vi "GetLIDARObstacles.vi"(11 "LIDAR data":cluster{"Magnitude":dbl[], "Direction":dbl[]}) -> (3 "LIDAR obstacles":cluster{dbl[], dbl[], i32})   [LabVIEW 2011]
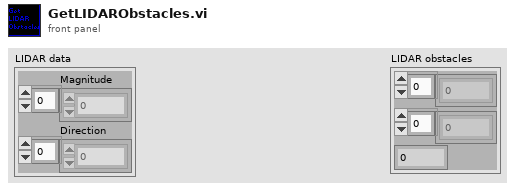
[diagram p1: front panel]
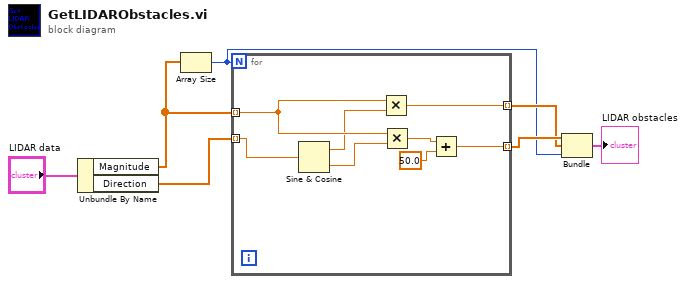
[diagram p0: block diagram]
diagram:
  n1 = Unbundle By Name("LIDAR data") -> ("Magnitude"=w7:dbl[], "Direction"=w6:dbl[])
  n2 = Array Size(array=w7) -> (size(s)=w3:i32)
  n3 = for {
    N: w3 -> [_]
    tunnel: w7 -> [w14] mode=indexing
    tunnel: w6 -> [w15] mode=indexing
    tunnel: [w11] -> w4 mode=indexing
    tunnel: [w8] -> w5 mode=indexing
    n4 = Sine & Cosine(0:w15) -> (1:w13:dbl, 2:w12:dbl)
    n5 = Multiply(x=w14, y=w13) -> (x*y=w11:dbl)
    n6 = Multiply(x=w14, y=w12) -> (x*y=w10:dbl)
    n7 = Add(x=w10, y=50.0) -> (x+y=w8:dbl)
  }
  n8 = Bundle(w5, w4, w3) -> (→"LIDAR obstacles":cluster{dbl[], dbl[], i32})  [unwired: 1 in]
